vi "F8588A Close.vi"(8 "error in (no error)":errorcluster, 11 "VISA resource name":refnum<visa-resource-name>) -> (0 "error out":errorcluster)   [LabVIEW 2020]
doc: "Performs an instrument error query before terminating the software connection to the instrument."
uses:
  <vilib>/Instr/_visa.llb/VISA GPIB Control REN Mode.ctl
  DMM/3458A Basic Driver/3458A Basic Driver.lvlib
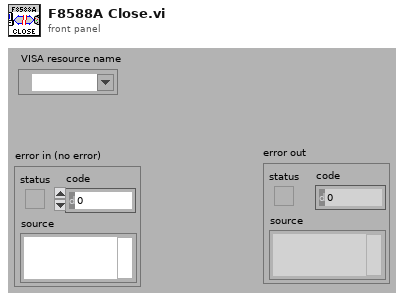
[diagram p1: front panel]
types:
  T1 = typedef "VISA GPIB Control REN Mode.ctl" = u16
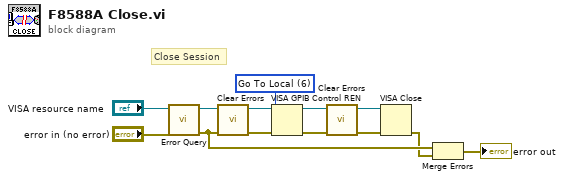
[diagram p0: block diagram]
diagram:
  w4 = T1 6 items=["Deassert REN", "Assert REN", "Go To Local; Deassert REN ", "Assert REN; Address Device", "Local Lockout (Addressed Devices)", "Local Lockout (This Device)", "Go To Local"] ("Mode")
  # "Close Session"
  n1 = call "Error Query.vi"("error in (no error)"="error in (no error)", "VISA resource name"="VISA resource name") -> ("error out"=w3:errorcluster, "VISA resource name out"=w6:refnum<visa-resource-name>)  [unwired: 6 in, 2 out]
  n2 = call <vilib>:"Clear Errors.vi"("error in (no error)"=w3) -> ("error out"=w8:errorcluster)  [unwired: 5 in, 1 out]
  n3 = VISA GPIB Control REN(8:w8, 10:w4, 11:w6) -> (0:w7:errorcluster, 3:w5:refnum<visa-resource-name>)
  n4 = call <vilib>:"Clear Errors.vi"("error in (no error)"=w7) -> ("error out"=w9:errorcluster)  [unwired: 5 in, 1 out]
  n5 = VISA Close(VISA resource name=w5, error in (no error)=w9) -> (error out=w2:errorcluster)
  n6 = Merge Errors(w3, w2) -> (→"error out":errorcluster)
